vi "Analyze LMS Data.vi"(1 "LMS Information Cluster In":T2) -> (0 "LMS Information Cluster Out":T1)   [LabVIEW 2014]
panel:
  out "LMS Vector Check":dbl[](array[numeric])
  out "Test SW Map Out of y":dbl[](array[numeric])
  out "Test SW Map Out of x":dbl[](array[numeric])
  # "Inputs:"
  # "Outputs:"
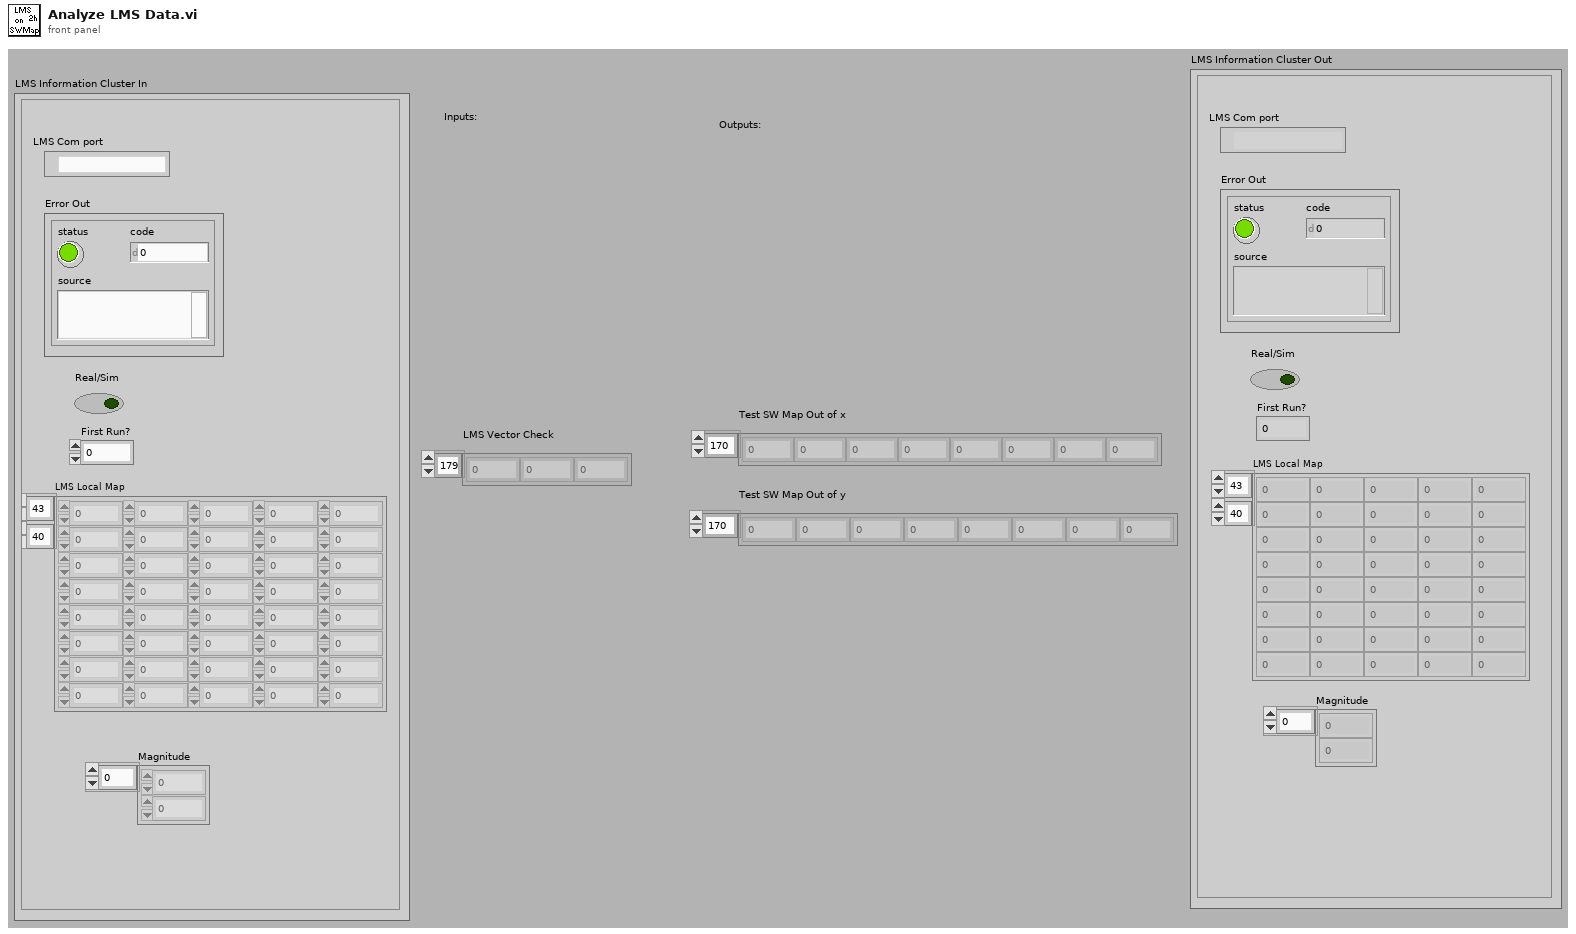
[diagram p1: front panel]
types:
  T1 = cluster{"LMS Com port":refnum<visa-resource-name>, "Error Out":errorcluster, "Real/Sim":bool, "First Run?":i32, "LMS Local Map ":dbl[][], "Magnitude":dbl[]}
  T2 = cluster{"LMS Com port":refnum<visa-resource-name>, "Error Out":errorcluster, "Real/Sim":bool, "First Run?":i32, "LMS Local Map ":i32[][], "Magnitude":dbl[]}
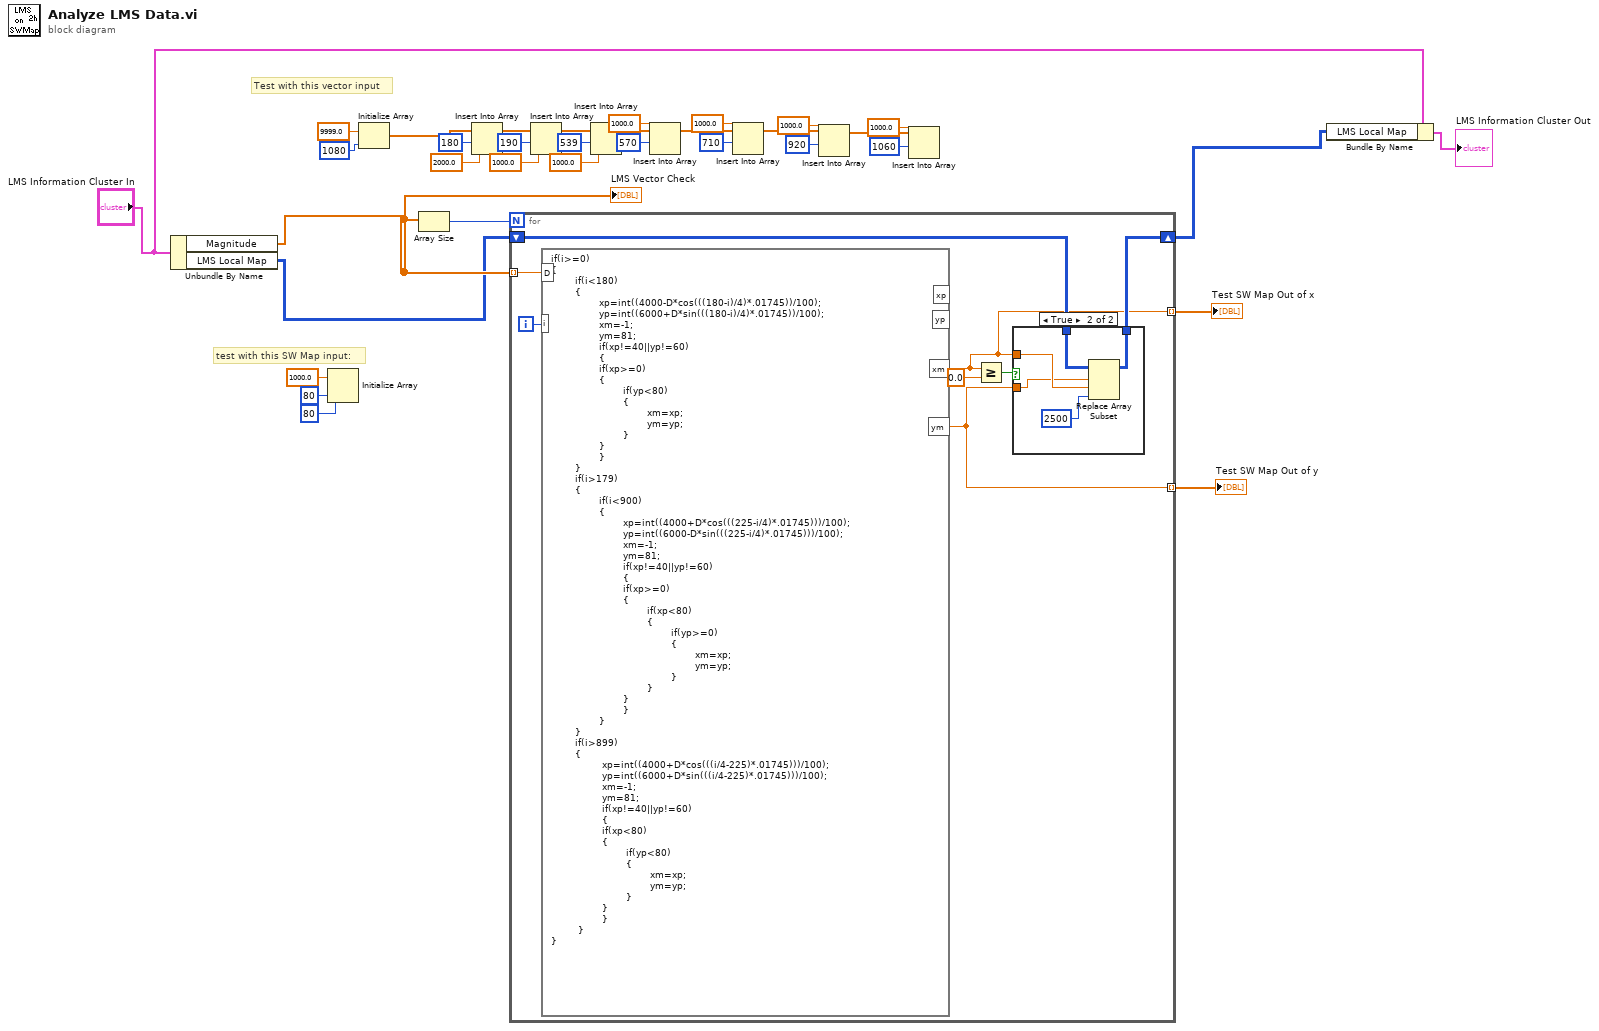
[diagram p0: block diagram]
diagram:
  # "test with this SW Map input:"
  # "Test with this vector input"
  n1 = Unbundle By Name("LMS Information Cluster In") -> ("Magnitude"=w5:dbl[], "LMS Local Map"=w4:i32[][])
  "LMS Vector Check" <- w5
  n2 = Initialize Array(1000.0 ("element"), 80 ("dimension size"), 80 ("dimension size")) -> ()  [unwired: 1 out]
  n3 = Initialize Array(9999.0 ("element"), 1080 ("dimension size")) -> (w33:dbl[])
  n4 = Array Size(array=w5) -> (size(s)=w31:i32)
  n5 = Insert Into Array(array=w33, index=180 ("index (row)"), new element=2000.0 ("new element/subarray")) -> (w6:dbl[])
  n6 = for {
    N: w31 -> [_]
    tunnel: w5 -> [w42] mode=indexing
    shift-right: [w37] -> w2
    shift-left: w4 -> [w40]
    tunnel: [w36] -> w11 mode=indexing
    tunnel: [w35] -> w10 mode=indexing
    i -> [w41]
    n7 = formula code="if(i>=0) \n{\n        if(i<180)\n        {\n                xp=int((4000-D*cos(((180-i)/4)*.01745))/100);\n                yp=int((6000+D*sin(((180-i)/4)*.01745))/100);\n                xm=-1;\n                ym=81;\n                if(xp!=40||yp!=60)\n                {\n                if(xp>=0)\n                {\n                        if(yp<80)\n                        {\n                                xm=xp;\n                                ym=yp;\n                        }\n                }\n                }\n        }\n        if(i>179)\n        {\n                if(i<900)\n                {\n                        xp=int((4000+D*cos(((225-i/4)*.01745)))/100);\n                        yp=int((6000-D*sin(((225-i/4)*.01745)))/100);\n                        xm=-1;\n                        ym=81;\n                        if(xp!=40||yp!=60)\n                        {\n                        if(xp>=0)\n                        {\n                                if(xp<80)\n                                {\n                                        if(yp>=0)\n                                        {\n                                                xm=xp;\n                                                ym=yp;\n                                        }\n                                }\n                        }\n                        }\n                }\n        }\n        if(i>899)\n        {\n                 xp=int((4000+D*cos(((i/4-225)*.01745)))/100);\n                 yp=int((6000+D*sin(((i/4-225)*.01745)))/100);\n                 xm=-1;\n                 ym=81;\n                 if(xp!=40||yp!=60)\n                 {\n                 if(xp<80)\n                 {\n                         if(yp<80)\n                         {\n                                 xm=xp;\n                                 ym=yp;\n                         }\n                 }\n                 }\n         }\n}"("D"=w42, "i"=w41) -> ("xm"=w35:dbl, "ym"=w36:dbl)  [unwired: 2 out]
    n8 = Greater Or Equal?(x=w35, y=0.0) -> (x >= y?=w38:bool)
    n9 = case shown="True" w38 {
      tunnel: w40 -> [w43 w48]
      tunnel: [w43 w47] -> w37
      tunnel: w36 -> [_ w44]
      tunnel: w35 -> [_ w45]
      frame False {
      }
      frame True {
        n10 = Replace Array Subset(array=w48, new element=2500, index (row)=w44, index (col)=w45) -> (w47:i32[][])
      }
    }
  }
  "Test SW Map Out of x" <- w10
  "Test SW Map Out of y" <- w11
  n11 = Insert Into Array(array=w6, index=190, new element=1000.0 ("new element/subarray")) -> (w26:dbl[])
  n12 = Insert Into Array(array=w26, index=539, new element=1000.0 ("new element/subarray")) -> (w23:dbl[])
  n13 = Insert Into Array(array=w23, index=570, new element=1000.0 ("new element/subarray")) -> (w20:dbl[])
  n14 = Insert Into Array(array=w20, index=710, new element=1000.0 ("new element/subarray")) -> (w17:dbl[])
  n15 = Insert Into Array(array=w17, index=920, new element=1000.0 ("new element/subarray")) -> (w14:dbl[])
  n16 = Insert Into Array(array=w14, index=1060, new element=1000.0 ("new element/subarray")) -> ()  [unwired: 1 out]
  n17 = Bundle By Name(cluster="LMS Information Cluster In", "LMS Local Map"=w2) -> (→"LMS Information Cluster Out":T2)
